vi "Waveform - Index Array.vi"() -> ()   [LabVIEW 2023]
doc: "Shows how to remove a single waveform from an array of waveforms."
uses:
  <vilib>/Waveform/WDTOps.llb/WDT Index Channel DBL.vi
panel:
  out "Selected Waveform":waveform(dbl)(graph)
  in  "Index":i32 min=0 max=2 step=1
  out "Initial Waveforms":waveform(dbl)[](graph)
  # "Overview: Demonstrates how to index individual waveforms out of a waveform array with the Index Waveform Array VI.\nInstructions:\n1. Select an Index value.\n2. Run the VI. The waveform at the specified Index will be displayed in the Selected Waveform graph."
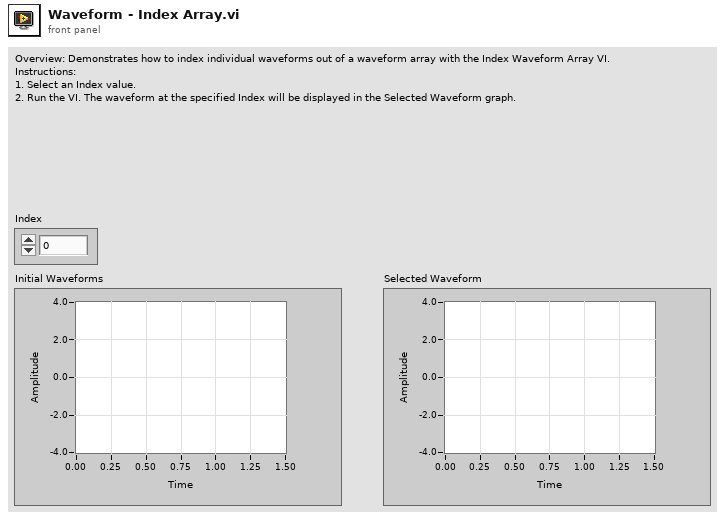
[diagram p1: front panel]
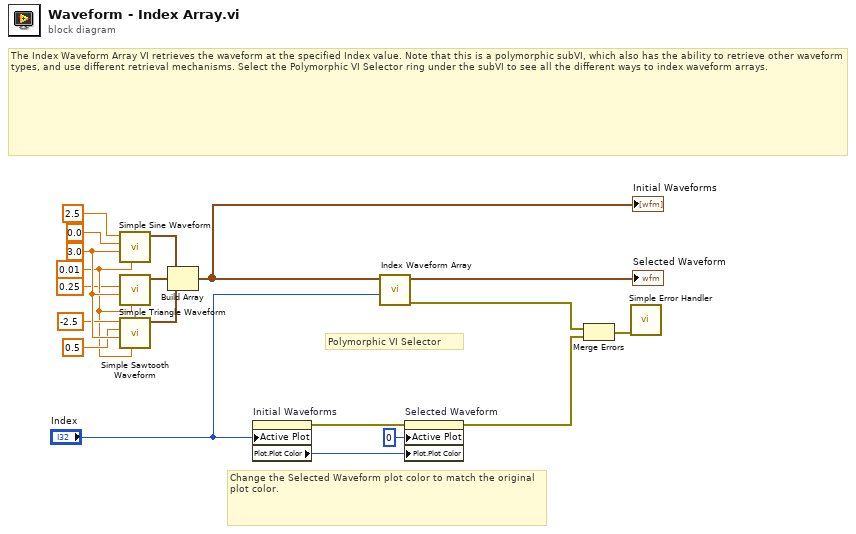
[diagram p0: block diagram]
diagram:
  w12 = 0.01
  w15 = 3.0
  # "Polymorphic VI Selector"
  # "Change the Selected Waveform plot color to match the original plot color."
  # "The Index Waveform Array VI retrieves the waveform at the specified Index value. Note that this is a polymorphic subVI, which also has the ability to retrieve other waveform types, and use different retrieval mechanisms. Select the Polymorphic VI Selector ring under the subVI to see all the different ways to index waveform arrays."
  n1 = call "Simple Sine Waveform.vi"("delta t"=w12, "n cycles"=w15, "t0"=0.0, "offset"=2.5) -> ("sine waveform"=w19:waveform(dbl))  [unwired: 7 in]
  n2 = call "Simple Triangle Waveform.vi"("delta t"=w12, "n cycles"=w15, "t0"=0.25) -> ("triangle waveform"=w18:waveform(dbl))  [unwired: 8 in]
  n3 = call "Simple Sawtooth Waveform.vi"("delta t"=w12, "n cycles"=w15, "t0"=0.5, "offset"=-2.5) -> ("sawtooth waveform"=w17:waveform(dbl))  [unwired: 7 in]
  n4 = Build Array(w19, w18, w17) -> (w7:waveform(dbl)[])
  "Initial Waveforms" <- w7
  n5 = property on="Initial Waveforms" class="WFGraph (strict)"("Active Plot"="Index") -> (error out=w4:errorcluster, "Plot.Plot Color"=w5:u32)  [unwired: 2 in, 1 out]
  n6 = call-poly <vilib>:"Index Waveform Array.vi"("index"="Index", "waveform array"=w7) -> ("error out"=w11:errorcluster, "waveform"=→"Selected Waveform":waveform(dbl))  [unwired: 8 in]
  n7 = property on="Selected Waveform" class="WFGraph (strict)"(error in=w4, "Active Plot"=u32 0, "Plot.Plot Color"=w5) -> (error out=w8:errorcluster)  [unwired: 1 in, 1 out]
  n8 = Merge Errors(w11, w8) -> (w10:errorcluster)
  n9 = call <vilib>:"Simple Error Handler.vi"("error in (no error)"=w10) -> ()  [unwired: 4 in, 5 out]
